vi "SelectCurve.vi"(1 "Mouse Position":cluster{"X":i32, "Y":i32}, 2 "Display State In":T1 caption="State") -> (0 "MinDistanceID":u8)   [LabVIEW 2016, in "FalseColorEditer.xctl"]
uses:
  FalseColorEditer.xctl
  State.ctl
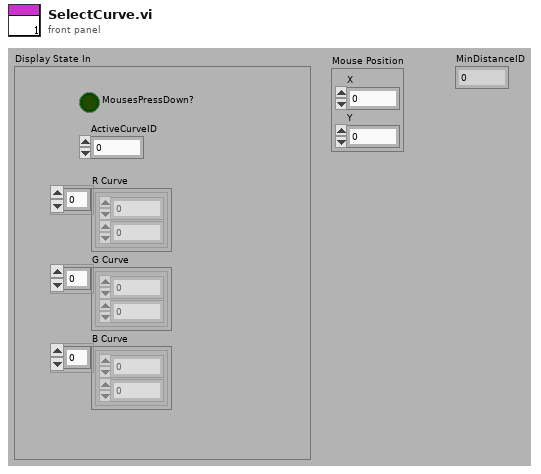
[diagram p1: front panel]
types:
  T1 = typedef "FalseColorEditer.xctl/State.ctl" = cluster{"MousesPressDown?":bool, "ActiveCurveID":i8, "R Curve ":cluster{i16, i16}[], "G Curve":cluster{i16, i16}[], "B Curve":cluster{i16, i16}[]}
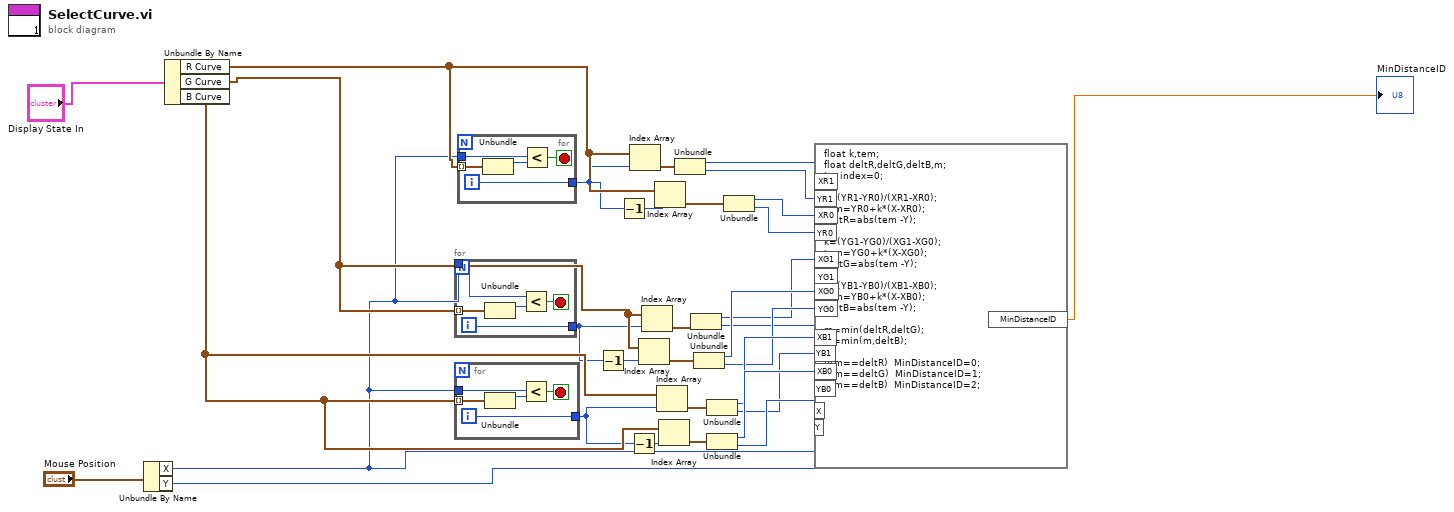
[diagram p0: block diagram]
diagram:
  n1 = Unbundle By Name("Mouse Position") -> ("X"=w22:i32, "Y"=w31:i32)
  n2 = Unbundle By Name("Display State In") -> ("R Curve"=w27:cluster{i16, i16}[], "G Curve"=w32:cluster{i16, i16}[], "B Curve"=w28:cluster{i16, i16}[])
  n3 = for {
    tunnel: w32 -> [w36] mode=indexing
    tunnel: w22 -> [w35]
    tunnel: [w37] -> w13
    i -> [w37]
    stop <- w33 stop-if-true
    n4 = Unbundle(w36) -> (w34:i16)  [unwired: 1 out]
    n5 = Less?(x=w35, y=w34) -> (x < y?=w33:bool)
  }
  n6 = for {
    tunnel: w28 -> [w41] mode=indexing
    tunnel: w22 -> [w40]
    tunnel: [w42] -> w18
    i -> [w42]
    stop <- w38 stop-if-true
    n7 = Unbundle(w41) -> (w39:i16)  [unwired: 1 out]
    n8 = Less?(x=w40, y=w39) -> (x < y?=w38:bool)
  }
  n9 = for {
    tunnel: w27 -> [w46] mode=indexing
    tunnel: w22 -> [w45]
    tunnel: [w47] -> w1
    i -> [w47]
    stop <- w43 stop-if-true
    n10 = Unbundle(w46) -> (w44:i16)  [unwired: 1 out]
    n11 = Less?(x=w45, y=w44) -> (x < y?=w43:bool)
  }
  n12 = Decrement(x=w13) -> (x-1=w12:i32)
  n13 = Decrement(x=w1) -> (x-1=w2:i32)
  n14 = Decrement(x=w18) -> (x-1=w19:i32)
  n15 = Index Array(array=w27, index=w1) -> (element=w4:cluster{i16, i16})
  n16 = Index Array(array=w32, index=w12) -> (element=w11:cluster{i16, i16})
  n17 = Index Array(array=w32, index=w13) -> (element=w10:cluster{i16, i16})
  n18 = Index Array(array=w27, index=w2) -> (element=w3:cluster{i16, i16})
  n19 = Index Array(array=w28, index=w18) -> (element=w21:cluster{i16, i16})
  n20 = Index Array(array=w28, index=w19) -> (element=w20:cluster{i16, i16})
  n21 = Unbundle(w4) -> (w8:i16, w9:i16)
  n22 = Unbundle(w10) -> (w14:i16, w15:i16)
  n23 = Unbundle(w11) -> (w16:i16, w17:i16)
  n24 = Unbundle(w21) -> (w23:i16, w24:i16)
  n25 = Unbundle(w20) -> (w26:i16, w25:i16)
  n26 = Unbundle(w3) -> (w6:i16, w7:i16)
  n27 = formula code="float k,tem;\nfloat deltR,deltG,deltB,m;\nint index=0;\n\nk=(YR1-YR0)/(XR1-XR0);\ntem=YR0+k*(X-XR0);\ndeltR=abs(tem -Y);\n\nk=(YG1-YG0)/(XG1-XG0);\ntem=YG0+k*(X-XG0);\ndeltG=abs(tem -Y);\n\nk=(YB1-YB0)/(XB1-XB0);\ntem=YB0+k*(X-XB0);\ndeltB=abs(tem -Y);\n\nm=min(deltR,deltG);\nm=min(m,deltB);\n\nif(m==deltR)  MinDistanceID=0; \nif(m==deltG)  MinDistanceID=1;\nif(m==deltB)  MinDistanceID=2;"("YR1"=w9, "XR1"=w8, "XR0"=w6, "YR0"=w7, "X"=w22, "Y"=w31, "XG1"=w14, "YG1"=w15, "XG0"=w16, "YG0"=w17, "XB1"=w23, "YB1"=w24, "XB0"=w26, "YB0"=w25) -> ("MinDistanceID"=→"MinDistanceID":dbl)
